vi "Cycle KnobTurn.vi"(8 "Error In":errorcluster, 10 "Cycle Knob":T2(ring), 11 "GEA2 Reference In":refnum<k24>) -> (0 "Error Out":errorcluster, 3 "GEA2 Reference Out":refnum<k24>)   [LabVIEW 2016, in "Centauro.lvlib"]
uses:
  Projects/Centauro.lvlib
  Q:/Common/DLLs/GEA3/GeaCommunication.dll
  Common/DLLs/GEA3/GeaCommunication.dll
  Tools/Laundry/Centauro Tool/Centauro Tool Support/type defs/Event Sequence.ctl
panel:
  in  "Event ID":T1
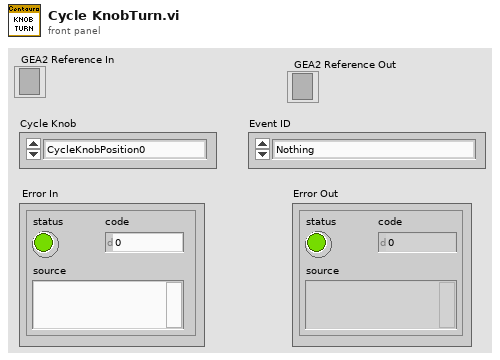
[diagram p1: front panel]
types:
  T1 = typedef "Event Sequence.ctl" = enum16{"Nothing", "StartButtonPress", "StartButtonRelease", "DeepRinseKeyPress", "DeepRinseKeyRelease", "CycleKnobPosition0", "CycleKnobPosition1", "CycleKnobPosition2", "CycleKnobPosition3", "CycleKnobPosition4", "CycleKnobPosition5", "CycleKnobPosition6", "CycleKnobPosition7", "CycleKnobPosition8", "CycleKnobPosition9", "CycleKnobPosition10", "CycleKnobPosition11", "OptionKnob1Position0", "OptionKnob1Position1", "OptionKnob1Position2", "OptionKnob1Position3", "OptionKnob1Position4", "OptionKnob1Position5", "OptionKnob2Position0", "OptionKnob2Position1", "OptionKnob2Position2", "OptionKnob2Position3", "OptionKnob2Position4"}
  T2 = enum16{"CycleKnobPosition0", "CycleKnobPosition1", "CycleKnobPosition2", "CycleKnobPosition3", "CycleKnobPosition4", "CycleKnobPosition5", "CycleKnobPosition6", "CycleKnobPosition7", "CycleKnobPosition8", "CycleKnobPosition9", "CycleKnobPosition10", "CycleKnobPosition11"}
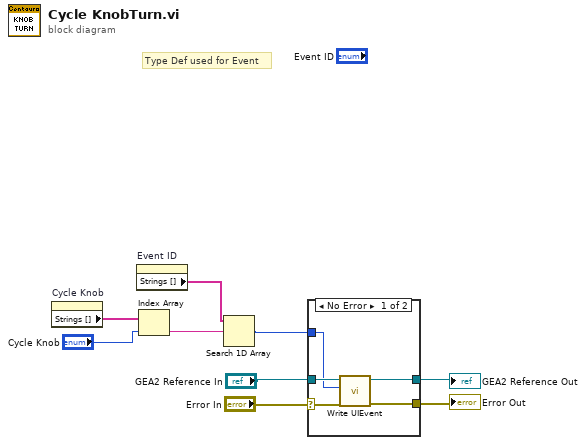
[diagram p0: block diagram]
diagram:
  # "Type Def used for Event"
  n1 = property on="Cycle Knob" class="Enum (strict)"() -> ("Strings []"=w4:string[])  [unwired: 2 in, 2 out]
  n2 = property on="Event ID" class="Enum (strict)"() -> ("Strings []"=w5:string[])  [unwired: 2 in, 2 out]
  n3 = Index Array(array=w4, index="Cycle Knob") -> (element=w6:string)
  n4 = Search 1D Array(1D array=w5, element=w6) -> (index of element=w2:i32)  [unwired: 1 in]
  n5 = case shown="No Error" "Error In" {
    selector: "Error In" -> [w13 w16]
    tunnel: [w14 w16] -> w1
    tunnel: "GEA2 Reference In" -> [w12 w15]
    tunnel: [w11 w15] -> w7
    tunnel: w2 -> [w10 _]
    frame No Error {
      n6 = call "Write UIEvent.vi"("Error In"=w13, "Event ID"=w10, "GEA2 Reference In"=w12) -> ("Error Out"=w14:errorcluster, "GEA2 Reference Out"=w11:refnum<k24>)  [unwired: 7 in]
    }
    frame Error {
    }
  }
  "Error Out" <- w1
  "GEA2 Reference Out" <- w7
